vi "Get Reg values from OPC.vi"(8 "error in (no error)":errorcluster, 9 "node IDs":T1, 10 "OPC UA client refnum in":T3, 11 "Regs_State in":T6(array[cluster]) {"Y_State"."Y" format="%.2f"; "Y_State"."Y_preSet" format="%.2f"; "Y_State"."SP" step=0.01 format="%.2f"; "Y_State"."Y_Set" format="%.2f"; "Y_State"."PV" step=0.01 format="%.2f"; "Y_State"."SP_Set" step=0.01 format="%.2f"}) -> (0 "error out":errorcluster, 3 "Regs_State out":T6(array[cluster]) {"Y_State"."Y" format="%.2f"; "Y_State"."Y_preSet" format="%.2f"; "Y_State"."SP" step=0.01 format="%.2f"; "Y_State"."Y_Set" format="%.2f"; "Y_State"."PV" step=0.01 format="%.2f"; "Y_State"."SP_Set" step=0.01 format="%.2f"})   [LabVIEW 2019, in "control.lvlib"]
uses:
  ctl/Y_short.ctl
  Inputs/Ctl/Parameter State short.ctl
  <vilib>/OPCUA/controls/OPC UA Client Refnum.ctl
  <vilib>/OPCUA/controls/NodeIds.ctl
  <vilib>/OPCUA/controls/NodeId.ctl
  b9864d16-88e2-443e-bd35-c8d49589a991.vi
  <vilib>/OPCUA/client/Multiple Read String.vi
  <vilib>/JDP Science/JSONtext/JSON text to Variant.vi
  <vilib>/JDP Science/JSONtext/LVClass Serializer/JSONtext LVClass Serializer.lvclass
  control.lvlib
  Inputs/Inputs.lvlib
  <vilib>/OPCUA/NI OPC UA Client.lvlib
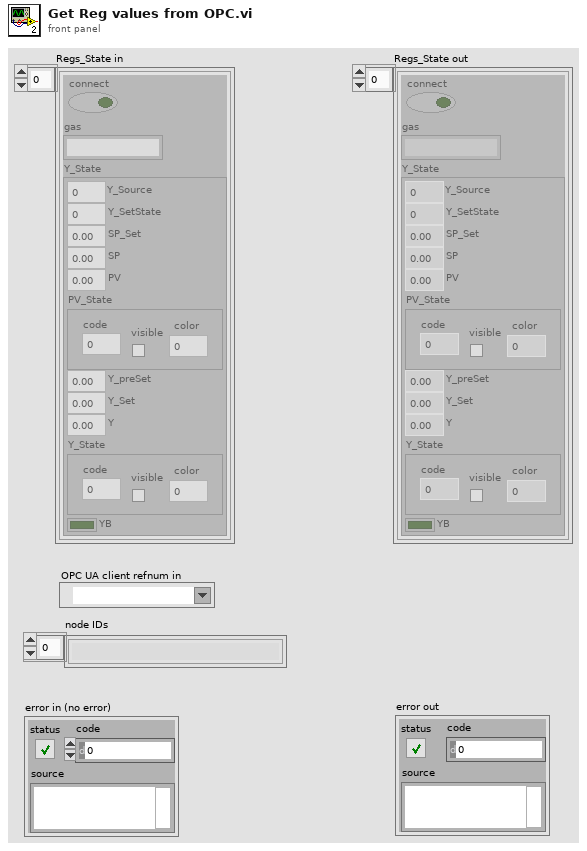
[diagram p1: front panel]
types:
  T1 = typedef "NodeIds.ctl" = T2[]
  T2 = typedef "NodeId.ctl" = string
  T3 = typedef "OPC UA Client Refnum.ctl" = refnum<k21>
  T4 = typedef "control.lvlib/Y_short.ctl" = cluster{"Y_Source":u8, "Y_SetState":u8, "SP_Set":dbl, "SP":dbl, "PV":dbl, "PV_State":T5, "Y_preSet":dbl, "Y_Set":dbl, "Y":dbl, "Y_State":T5, "YB":bool}
  T5 = typedef "Inputs.lvlib/Parameter State short.ctl" = cluster{"code":i32, "visible":bool, "color":u32}
  T6 = cluster{"connect":bool, "gas":string, "Y_State":T4}[]
  T7 = typedef "OPC UA StatusCode.ctl" = u32
  T8 = cluster{"node ID":T2, "value ":string, "timestamp":timestamp, "status":T7}[]
  T9 = cluster{"connect":bool, "gas":string, "Y_State":T4}
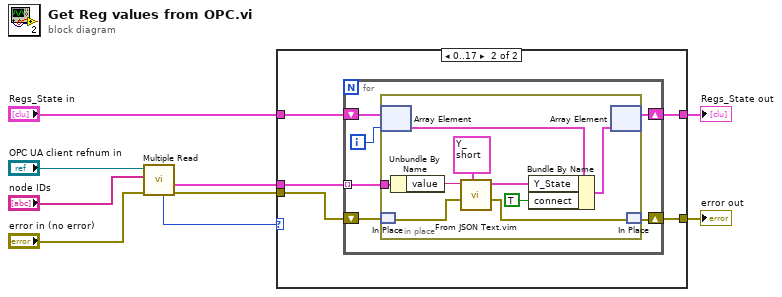
[diagram p0: block diagram]
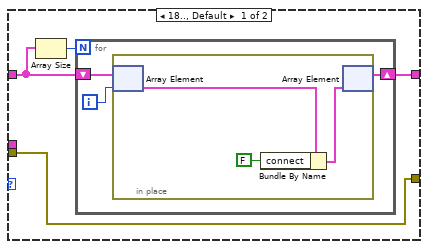
[diagram p2: hidden frame]
diagram:
  n1 = call-poly <vilib>:"Multiple Read.vi"("error in (no error)"="error in (no error)", "node IDs"="node IDs", "OPC UA client refnum in"="OPC UA client refnum in") -> ("error out"=w2:errorcluster, "results"=w3:T8, "service status"=w1:T7)  [unwired: 5 in, 1 out]
  n2 = case shown="0..17" w1 {
    tunnel: [w11 w24] -> w9
    tunnel: [w10 w23] -> w8
    tunnel: "Regs_State in" -> [w12 w22]
    tunnel: w3 -> [_ w21]
    tunnel: w2 -> [w10 w20]
    frame 18.., Default {
      n3 = Array Size(array=w12) -> (size(s)=w13:i32)
      n4 = for {
        N: w13 -> [_]
        shift-right: [w14] -> w11
        shift-left: w12 -> [w16]
        i -> [w15]
        n5 = in-place {
          n6 = in-place-array #1(w16, w15) -> (w18:T9)
          n7 = Bundle By Name(cluster=w18, "connect"=FALSE) -> (w17:T9)
          n8 = in-place-array #1(w17) -> (w14:T6)  [unwired: 1 out]
        }
      }
    }
    frame 0..17 {
      n9 = for {
        shift-right: [w26] -> w23
        shift-left: w20 -> [w27]
        shift-right: [w28] -> w24
        shift-left: w22 -> [w30]
        tunnel: w21 -> [w25] mode=indexing
        i -> [w29]
        n10 = in-place {
          in-place-border: w25 -> [w31]
          n11 = in-place-array #2(w30, w29) -> (w38:T9)
          n12 = in-place-match #3(w27) -> (w33:errorcluster)
          n13 = Unbundle By Name(w31) -> ("value"=w36:string)
          n14 = call "From JSON Text.vim"("Data Type and Default Value"=T4 {"Y_Source"=3, "Y_SetState"=0, "SP_Set"=0.0, "SP"=0.0, "PV"=0.0, "PV_State"={"code"=0, "visible"=FALSE, "color"=0}, "Y_preSet"=0.0, "Y_Set"=0.0, "Y"=0.0, "Y_State"={"code"=0, "visible"=FALSE, "color"=0}, "YB"=FALSE} ("Y_State"), "error in (no error)"=w33, "JSON"=w36) -> ("error out"=w32:errorcluster, "Data out"=w34:T4)  [unwired: 7 in]
          n15 = Bundle By Name(cluster=w38, "Y_State"=w34, "connect"=TRUE) -> (w37:T9)
          n16 = in-place-array #2(w37) -> (w28:T6)  [unwired: 1 out]
          n17 = in-place-match #3(w32) -> (w26:errorcluster)
        }
      }
    }
  }
  "Regs_State out" <- w9
  "error out" <- w8
